vi "Update SYMLINK conventions.vi"(10 "OpenSSH detected":bool, 11 "session in":refnum<class "Session.lvclass">) -> (3 "session out":refnum<class "Session.lvclass">)   [LabVIEW 2020, in "NI_SFTP.lvlib" / "Session.lvclass"]
uses:
  <vilib>/net/SFTP/Session/Session.lvclass
  <vilib>/net/SFTP/Session/Session.lvclass/Session.ctl
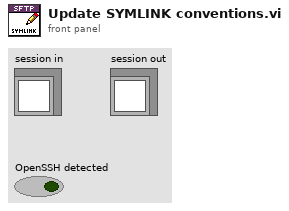
[diagram p1: front panel]
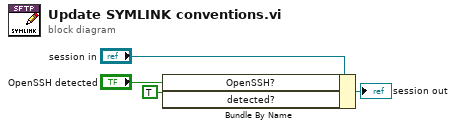
[diagram p0: block diagram]
diagram:
  n1 = Bundle By Name(cluster="session in", "OpenSSH?"="OpenSSH detected", "detected?"=TRUE ("SYMLINK convention.detected?")) -> (→"session out":refnum<class "Session.lvclass">)
